vi "AutoLauncher.vi"(11 "# Frisbees":i32) -> ()   [LabVIEW 2013]
uses:
  State_Machine_Enum.ctl
  Sally_Dashboard_2014/DBNameEnum.ctl
  Robot Global Data.vi
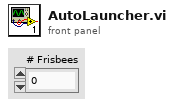
[diagram p1: front panel]
types:
  T1 = typedef "State_Machine_Enum.ctl" = enum16{"Idle", "Start", "Do", "Stop", "Init"}
  T2 = typedef "DBNameEnum.ctl" = enum16{"AutoInstructions", "DriveLoopTime", "DriveAlignLSLeft", "DriveAlignLSRight", "Use2DriveAlign", "ClimbLS", "LauncherAngleMatches", "FrameworkVersion", "sLauncherAngle", "LauncherTargetAngle", "sLauncherRPM", "LauncherTargetRPM", "sDriveDistance", "LauncherMotorValue", "PullbackTol", "FireTol", "LauncherRPMTol", "LauncherAngleTol", "InitialWait", "WaitBetweenLaunch", "AnglePresets", "RPMPresets", "UseAngleEncoder", "UseLauncherEncoder", "UseLauncherPID", "QSWaitBeforeFire", "QSWaitBeforeRetract", "AngleForwardValue", "AngleBackwardValue", "UseClusterArray", "BackupAuto", "ReverseDriveIndicate", "HalfSpeedFactor"}
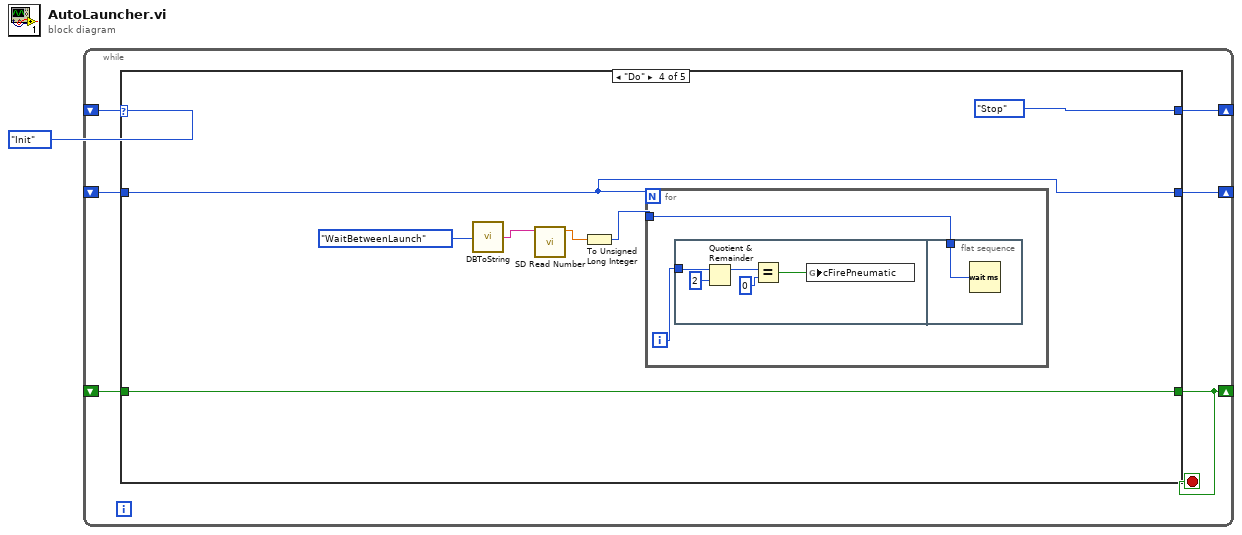
[diagram p0: block diagram]
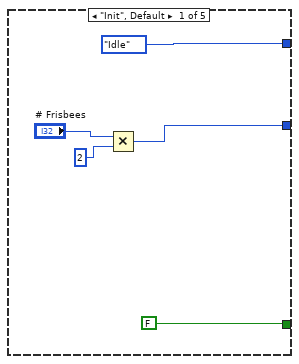
[diagram p2: hidden frame]
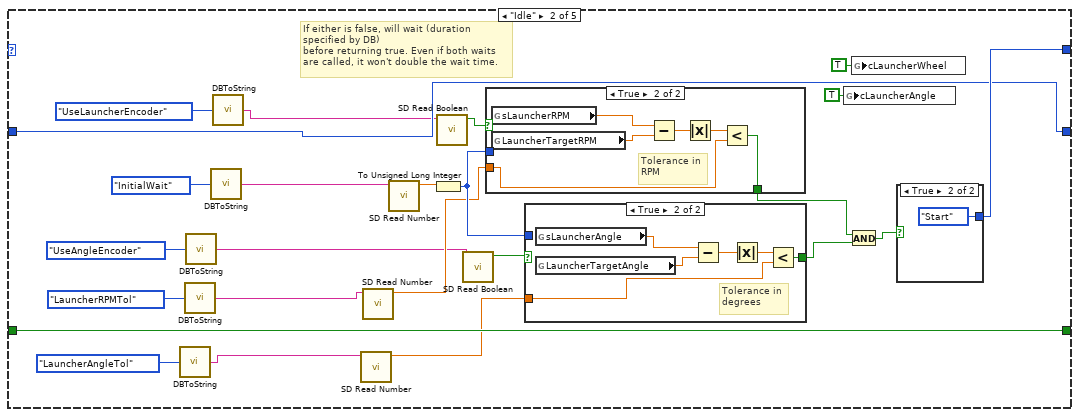
[diagram p3: hidden frame]
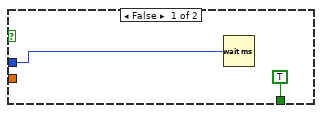
[diagram p4: hidden frame]
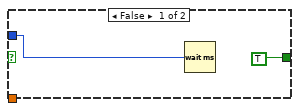
[diagram p5: hidden frame]
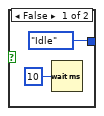
[diagram p6: hidden frame]
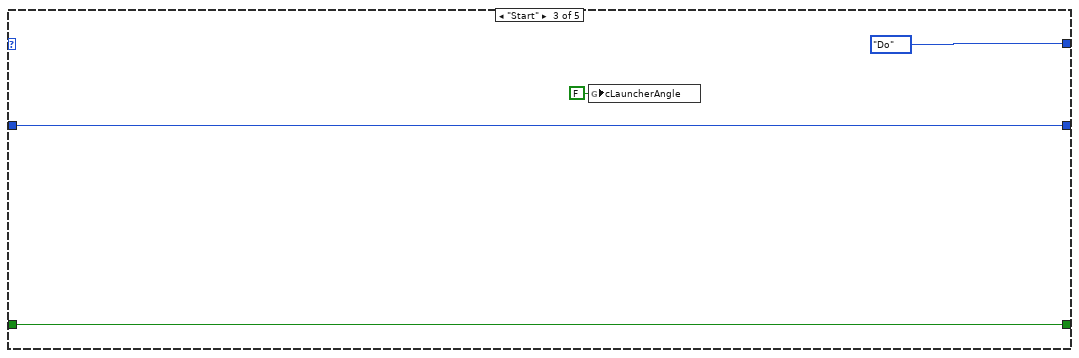
[diagram p7: hidden frame]
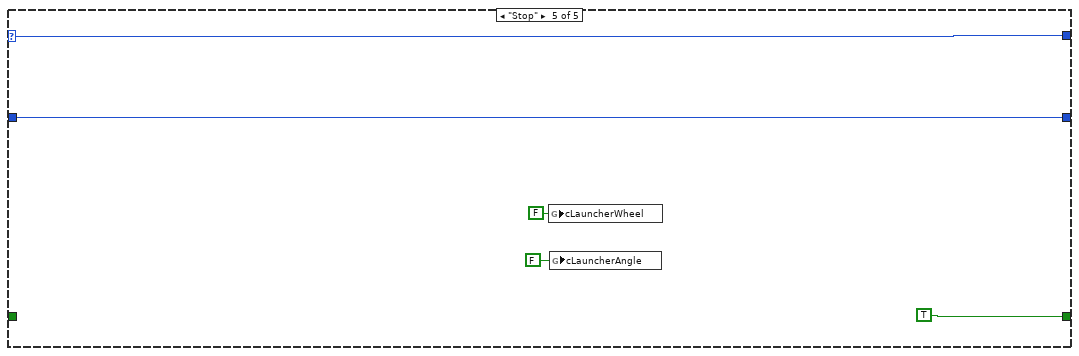
[diagram p8: hidden frame]
diagram:
  n1 = while {
    shift-right: [w6] -> _
    shift-left: State_Machine_Enum."Init" ("State") -> [w7]
    shift-right: [w5] -> _
    shift-left: _ -> [w4]
    shift-right: [w3] -> _
    shift-left: _ -> [w2]
    stop <- w5 stop-if-true
    n2 = case shown="\"Do\"" w7 {
      selector: w7 -> [_ _ _ _ w77]
      tunnel: [State_Machine_Enum."Idle" ("State") w33 State_Machine_Enum."Do" ("State") State_Machine_Enum."Stop" ("State") w77] -> w6
      tunnel: [FALSE w36 w58 w65 TRUE] -> w5
      tunnel: w4 -> [_ w36 w58 w65 _]
      tunnel: [w8 w32 w57 w66 w78] -> w3
      tunnel: w2 -> [_ w32 w57 w66 w78]
      frame "Init", Default {
        n3 = Multiply(x="# Frisbees", y=2) -> (x*y=w8:i32)
      }
      frame "Idle" {
        # "If either is false, will wait (duration specified by DB)\nbefore returning true. Even if both waits are called, it won't double the wait time."
        n4 = call "DBToString.vi"("Enum"=DBNameEnum."LauncherAngleTol") -> ("Refname"=w17:string)
        n5 = call "DBToString.vi"("Enum"=DBNameEnum."LauncherRPMTol") -> ("Refname"=w16:string)
        n6 = call "DBToString.vi"("Enum"=DBNameEnum."UseAngleEncoder") -> ("Refname"=w15:string)
        n7 = call "DBToString.vi"("Enum"=DBNameEnum."InitialWait") -> ("Refname"=w14:string)
        n8 = call "DBToString.vi"("Enum"=DBNameEnum."UseLauncherEncoder") -> ("Refname"=w13:string)
        n9 = call <vilib>:"SD Read Number.vi"("Name"=w17) -> ("Numeric"=w23:dbl)  [unwired: 8 in, 2 out]
        n10 = call <vilib>:"SD Read Number.vi"("Name"=w16) -> ("Numeric"=w24:dbl)  [unwired: 8 in, 2 out]
        n11 = call <vilib>:"SD Read Number.vi"("Name"=w14) -> ("Numeric"=w26:dbl)  [unwired: 8 in, 2 out]
        n12 = To Unsigned Long Integer(number=w26) -> (unsigned 32bit integer=w25:u32)
        n13 = call <vilib>:"SD Read Boolean.vi"("Name"=w13) -> ("Boolean"=w27:bool)  [unwired: 8 in, 2 out]
        n14 = call <vilib>:"SD Read Boolean.vi"("Name"=w15) -> ("Boolean"=w28:bool)  [unwired: 8 in, 2 out]
        n15 = case shown="True" w27 {
          tunnel: [TRUE w44] -> w35
          tunnel: w25 -> [w37 _]
          tunnel: w24 -> [_ w39]
          frame False {
            n16 = Wait (ms)(milliseconds to wait=w37) -> ()  [unwired: 1 out]
          }
          frame True {
            # "Tolerance in\nRPM"
            n17 = global read "Robot Global Data.vi" "sLauncherRPM"() -> (w43:dbl)
            n18 = global read "Robot Global Data.vi" "LauncherTargetRPM"() -> (w42:dbl)
            n19 = Subtract(x=w43, y=w42) -> (x-y=w41:dbl)
            n20 = Absolute Value(x=w41) -> (abs(x)=w40:dbl)
            n21 = Less?(x=w40, y=w39) -> (x < y?=w44:bool)
          }
        }
        n22 = case shown="True" w28 {
          tunnel: [TRUE w48] -> w29
          tunnel: w25 -> [w45 _]
          tunnel: w23 -> [_ w47]
          frame False {
            n23 = Wait (ms)(milliseconds to wait=w45) -> ()  [unwired: 1 out]
          }
          frame True {
            # "Tolerance in\ndegrees"
            n24 = global read "Robot Global Data.vi" "sLauncherAngle"() -> (w49:dbl)
            n25 = global read "Robot Global Data.vi" "LauncherTargetAngle"() -> (w50:dbl)
            n26 = Subtract(x=w49, y=w50) -> (x-y=w51:dbl)
            n27 = Absolute Value(x=w51) -> (abs(x)=w52:dbl)
            n28 = Less?(x=w52, y=w47) -> (x < y?=w48:bool)
          }
        }
        n29 = global write "Robot Global Data.vi" "cLauncherAngle"(TRUE ("cLauncherAngle")) -> ()
        n30 = And(x=w35, y=w29) -> (x .and. y?=w34:bool)
        n31 = global write "Robot Global Data.vi" "cLauncherWheel"(TRUE ("cLauncherWheel")) -> ()
        n32 = case shown="True" w34 {
          tunnel: [State_Machine_Enum."Idle" ("State") State_Machine_Enum."Start" ("State")] -> w33
          frame False {
            n33 = Wait (ms)(milliseconds to wait=u32 10) -> ()  [unwired: 1 out]
          }
          frame True {
          }
        }
      }
      frame "Start" {
        n34 = global write "Robot Global Data.vi" "cLauncherAngle"(FALSE ("cLauncherAngle")) -> ()
      }
      frame "Do" {
        n35 = call "DBToString.vi"("Enum"=DBNameEnum."WaitBetweenLaunch") -> ("Refname"=w60:string)
        n36 = call <vilib>:"SD Read Number.vi"("Name"=w60) -> ("Numeric"=w63:dbl)  [unwired: 8 in, 2 out]
        n37 = To Unsigned Long Integer(number=w63) -> (unsigned 32bit integer=w62:u32)
        n38 = for {
          N: w66 -> [_]
          tunnel: w62 -> [w67]
          i -> [w68]
          n39 = flat-sequence {
            tunnel: w68 -> [w73]
            tunnel: w67 -> [w74]
            frame #0 {
              n40 = Quotient & Remainder(x=w73, y=2) -> (x-y*floor(x/y)=w71:i32)  [unwired: 1 out]
              n41 = Equal?(x=w71, y=0) -> (x = y?=w69:bool)
              n42 = global write "Robot Global Data.vi" "cFirePneumatic"(w69) -> ()
            }
            frame #1 {
              n43 = Wait (ms)(milliseconds to wait=w74) -> ()  [unwired: 1 out]
            }
          }
        }
      }
      frame "Stop" {
        n44 = global write "Robot Global Data.vi" "cLauncherWheel"(FALSE ("cLauncherWheel")) -> ()
        n45 = global write "Robot Global Data.vi" "cLauncherAngle"(FALSE ("cLauncherWheel")) -> ()
      }
    }
  }
